vi "generate_DAC_voltages_original.vi"(7 "focus mode?":bool, 8 "derived values":T1, 9 "scan specification":T4={"x amplitude"=0, "x resolution (pixels)"=0, "x offset fly-forward (iterations)"=0, "x offset fly-back (iterations)"=0, "y resolution (nr. of lines)"=0, "y step size"=0, "iterations per pixel"=0, "number of frames"=0, "y offset (pixels)"=0, "number of y-brake lines  (before y-fly-back)"=0, "number y-brake lines (after y-fly-back)"=0, "number of y-fly-back steps"=8, "lines per z step"=0, "number of z/intensity tuples"=0, "number of repetitions (volumes or planes)"=0, "z step size derived"=0, "choose the beginning of z scan"=FALSE, "number of frames (settings)"=0, "FPGA trajectory?"=FALSE}, 10 "counter cluster in":T2, 11 "resonant trigger":bool) -> (0 "acquire?":bool, 1 "fly-back acquisition phase?":bool, 2 "counter cluster out":T2, 3 "DAC voltages":T3 {"ch6" max=4095 step=1; "ch5" max=4095 step=1; "ch4" max=4095 step=1; "ch3" max=4095 step=1; "ch2" max=4095 step=1; "ch1" max=4095 step=1; "ch0" max=4095 step=1})   [LabVIEW 2010]
uses:
  scan_specification_cluster.ctl
  common_typedefs/DAC_voltage_cluster.ctl
  counter_cluster.ctl
  derived_values_cluster.ctl
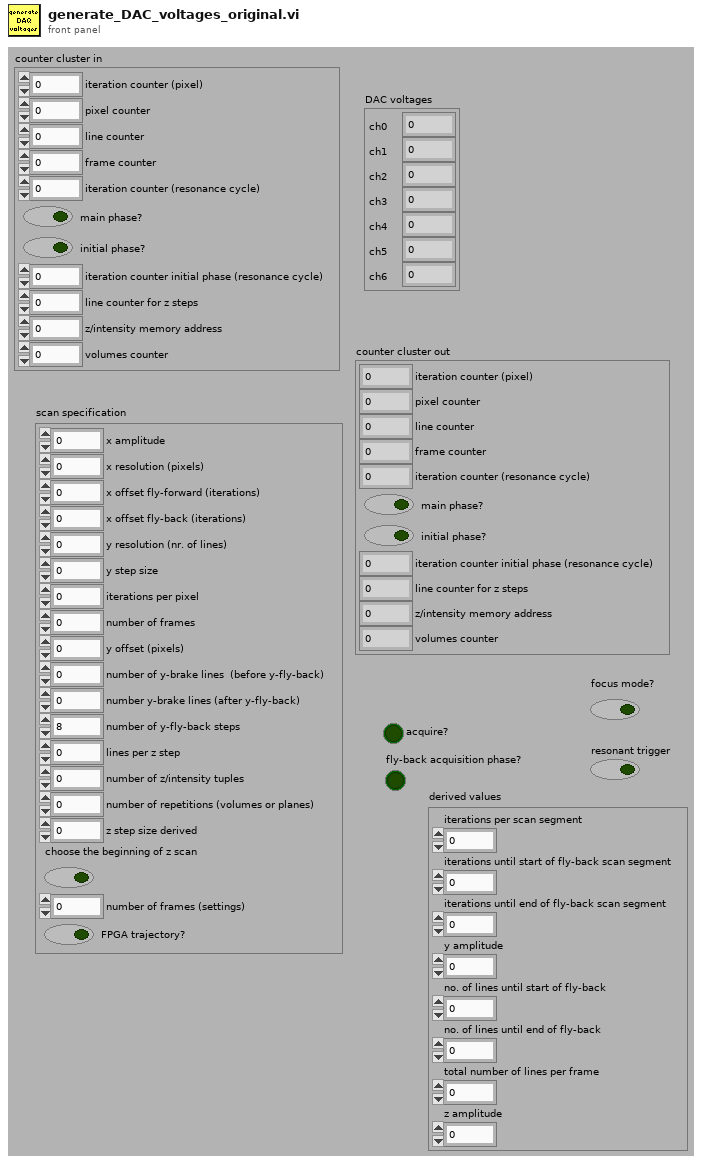
[diagram p1: front panel]
types:
  T1 = typedef "derived_values_cluster.ctl" = cluster{"iterations per scan segment":u16, "iterations until start of fly-back scan segment":u16, "iterations until end of fly-back scan segment":u16, "y amplitude":u16, "no. of lines until start of fly-back":u16, "no. of lines until end of fly-back":u16, "total number of lines per frame ":u16, "z amplitude":u16}
  T2 = typedef "counter_cluster.ctl" = cluster{"iteration counter (pixel)":u16, "pixel counter":u16, "line counter":u16, "frame counter":u16, "iteration counter (resonance cycle)":u16, "main phase?":bool, "initial phase?":bool, "iteration counter initial phase (resonance cycle)":u16, "line counter for z steps":u16, "z/intensity memory address":u32, "volumes counter":u16}
  T3 = typedef "DAC_voltage_cluster.ctl" = cluster{"ch0":u16, "ch1":i16, "ch2":i16, "ch3":u16, "ch4":u16, "ch5":u16, "ch6":u16}
  T4 = typedef "scan_specification_cluster.ctl" = cluster{"x amplitude":u16, "x resolution (pixels)":u16, "x offset fly-forward (iterations)":u16, "x offset fly-back (iterations)":u16, "y resolution (nr. of lines)":u16, "y step size":u16, "iterations per pixel":u16, "number of frames":i32, "y offset (pixels)":u16, "number of y-brake lines  (before y-fly-back)":u16, "number y-brake lines (after y-fly-back)":u16, "number of y-fly-back steps":u16, "lines per z step":u16, "number of z/intensity tuples":u16, "number of repetitions (volumes or planes)":i32, "z step size derived":u16, "choose the beginning of z scan":bool, "number of frames (settings)":i32, "FPGA trajectory?":bool}
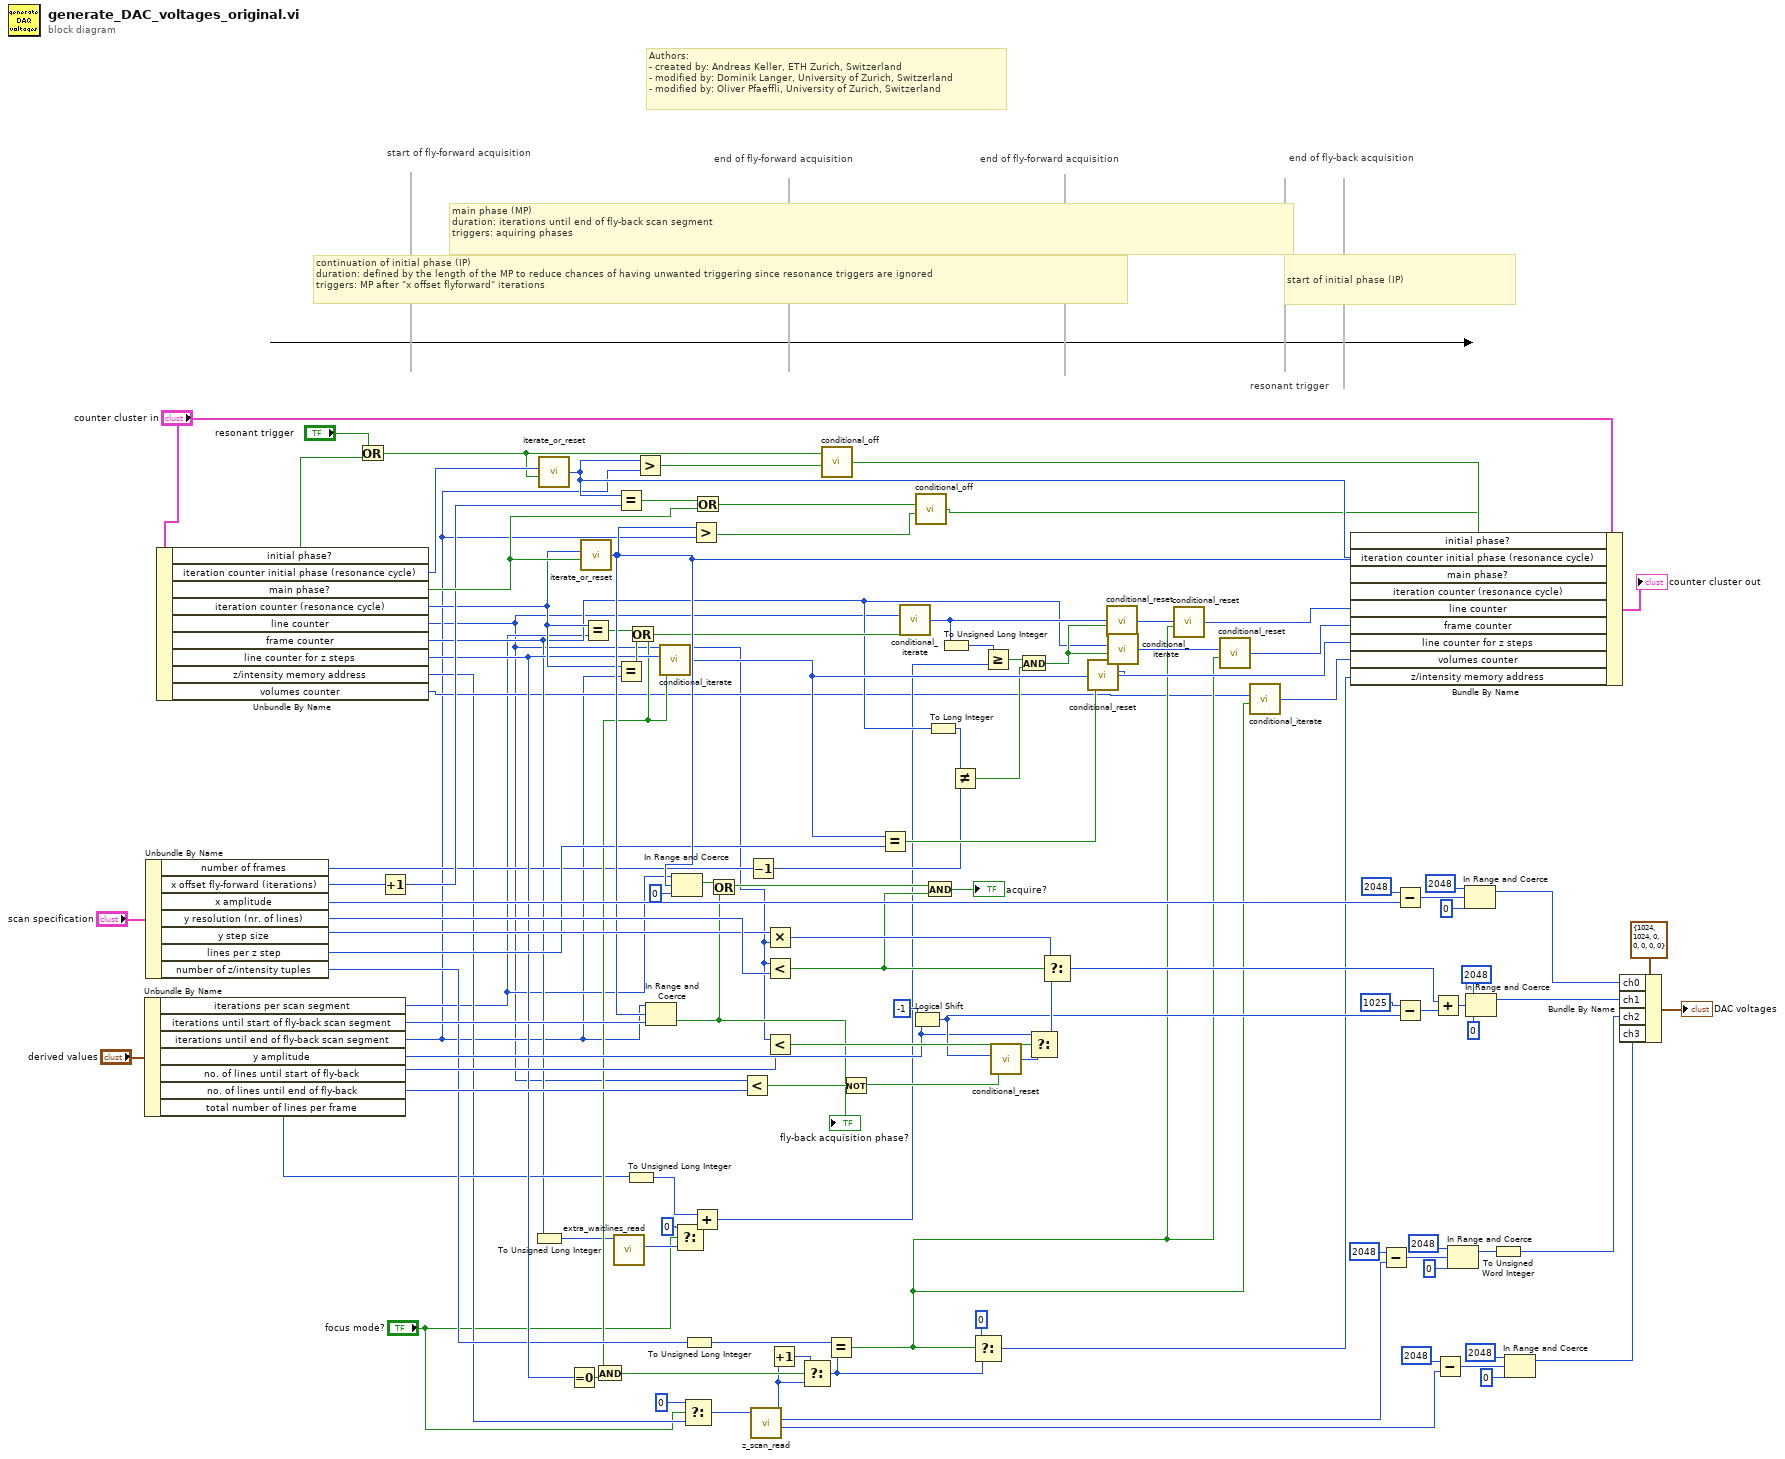
[diagram p0: block diagram]
diagram:
  # "start of initial phase (IP)"
  # "continuation of initial phase (IP)\nduration: defined by the length of the MP to reduce chances of having unwanted triggering since resonance triggers are ignored\ntriggers: MP after \"x offset flyforward\" iterations"
  # "end of fly-back acquisition"
  # "end of fly-forward acquisition"
  # "end of fly-forward acquisition"
  # "start of fly-forward acquisition"
  # "main phase (MP)\nduration: iterations until end of fly-back scan segment\ntriggers: aquiring phases"
  # "resonant trigger"
  # "Authors: \n- created by: Andreas Keller, ETH Zurich, Switzerland\n- modified by: Dominik Langer, University of Zurich, Switzerland\n- modified by: Oliver Pfaeffli, University of Zurich, Switzerland"
  n1 = Unbundle By Name("derived values") -> ("iterations per scan segment"=w5:u16, "iterations until start of fly-back scan segment"=w85:u16, "iterations until end of fly-back scan segment"=w4:u16, "y amplitude"=w69:u16, "no. of lines until start of fly-back"=w68:u16, "no. of lines until end of fly-back"=w84:u16, "total number of lines per frame"=w31:u16)
  n2 = Unbundle By Name("scan specification") -> ("number of frames"=w20:i32, "x offset fly-forward (iterations)"=w67:u16, "x amplitude"=w94:u16, "y resolution (nr. of lines)"=w91:u16, "y step size"=w90:u16, "lines per z step"=w59:u16, "number of z/intensity tuples"=w53:u16)
  n3 = Unbundle By Name("counter cluster in") -> ("initial phase?"=w83:bool, "iteration counter initial phase (resonance cycle)"=w80:u16, "main phase?"=w79:bool, "iteration counter (resonance cycle)"=w63:u16, "line counter"=w2:u16, "frame counter"=w17:u16, "line counter for z steps"=w55:u16, "z/intensity memory address"=w8:u32, "volumes counter"=w10:u16)
  n4 = Or(x="resonant trigger", y=w83) -> (x .or. y?=w76:bool)
  n5 = Increment(x=w67) -> (x+1=w66:u16)
  n6 = To Unsigned Long Integer(number=w17) -> (unsigned 32bit integer=w32:u32)
  n7 = call "iterate_or_reset.vi"("iterate?"=w76, "number in"=w80) -> ("number out"=w64:u16)  [unwired: 4 in]
  n8 = Equal To 0?(x=w55) -> (x = 0?=w38:bool)
  n9 = call "iterate_or_reset.vi"("iterate?"=w79, "number in"=w63) -> ("number out"=w78:u16)  [unwired: 4 in]
  n10 = Equal?(x=w63, y=w5) -> (x = y?=w60:bool)
  n11 = call "extra_waitlines_read.vi"("address extra waitlines IN"=w32) -> ("extra waitline data"=w13:u32)  [unwired: 9 in, 1 out]
  n12 = Equal?(x=w64, y=w66) -> (x = y?=w77:bool)
  n13 = Equal?(x=w63, y=w4) -> (x = y?=w62:bool)
  n14 = To Unsigned Long Integer(number=w31) -> (unsigned 32bit integer=w30:u32)
  n15 = Or(x=w60, y=w62) -> (x .or. y?=w37:bool)
  n16 = And(x=w37, y=w38) -> (x .and. y?=w36:bool)
  n17 = Greater?(x=w64, y=w4) -> (0:w65:bool)
  n18 = In Range and Coerce(upper limit=w4, x=w78, lower limit=w85) -> (In Range?=w61:bool)  [unwired: 1 out]
  "fly-back acquisition phase?" <- w61
  n19 = call "conditional_iterate.vi"("iterate?"=w37, "number in"=w55) -> ("number out"=w56:u16)  [unwired: 4 in]
  n20 = In Range and Coerce(upper limit=w5, x=w78, lower limit=u16 0) -> (In Range?=w106:bool)  [unwired: 1 out]
  n21 = Select(t=u32 0, s="focus mode?", f=w13) -> (s? t:f=w12:u32)
  n22 = Select(t=u32 0, s="focus mode?", f=w8) -> (s? t:f=w7:u32)
  n23 = To Unsigned Long Integer(number=w53) -> (unsigned 32bit integer=w52:u32)
  n24 = Greater?(x=w78, y=w4) -> (0:w74:bool)
  n25 = Add(x=w30, y=w12) -> (x+y=w14:u32)
  n26 = Or(x=w77, y=w79) -> (x .or. y?=w73:bool)
  n27 = Or(x=w106, y=w61) -> (x .or. y?=w89:bool)
  n28 = Less?(x=w2, y=w84) -> (x < y?=w87:bool)
  n29 = Decrement(x=w20) -> (x-1=w19:i32)
  n30 = call "z_scan_read.vi"("address in"=w7) -> ("intensity"=w35:u16, "z-value"=w33:i16, "address out"=w34:u32)  [unwired: 8 in]
  n31 = Multiply(x=w90, y=w2) -> (x*y=w112:u16)
  n32 = Less?(x=w2, y=w91) -> (x < y?=w88:bool)
  n33 = Less?(x=w2, y=w68) -> (x < y?=w114:bool)
  n34 = Increment(x=w34) -> (x+1=w54:u32)
  n35 = Select(t=w54, s=w36, f=w34) -> (s? t:f=w51:u32)
  n36 = call "conditional_off.vi"("switch off?"=w65, "boolean in"=w76) -> ("boolean out"=w75:bool)  [unwired: 4 in]
  n37 = Equal?(x=w52, y=w51) -> (x = y?=w15:bool)
  n38 = Not(x=w87) -> (.not. x?=w71:bool)
  n39 = Equal?(x=w56, y=w59) -> (x = y?=w57:bool)
  n40 = call "conditional_iterate.vi"("iterate?"=w37, "number in"=w2) -> ("number out"=w29:u16)  [unwired: 4 in]
  n41 = Logical Shift(y=i16 -1 ("n"), x=w69) -> (x << y=w72:u16)
  n42 = call "conditional_off.vi"("switch off?"=w74, "boolean in"=w73) -> ("boolean out"=w1:bool)  [unwired: 4 in]
  n43 = And(x=w89, y=w88) -> (x .and. y?=→"acquire?":bool)
  n44 = To Long Integer(number=w17) -> (32bit integer=w16:i32)
  n45 = To Unsigned Long Integer(number=w29) -> (unsigned 32bit integer=w28:u32)
  n46 = Not Equal?(x=w16, y=w19) -> (x != y?=w18:bool)
  n47 = Select(t=u32 0, s=w15, f=w51) -> (s? t:f=w27:u32)
  n48 = Greater Or Equal?(x=w28, y=w14) -> (x >= y?=w22:bool)
  n49 = call "conditional_reset.vi"("reset?"=w71, "number in"=w72) -> ("number out"=w70:u16)  [unwired: 4 in]
  n50 = And(x=w22, y=w18) -> (x .and. y?=w21:bool)
  n51 = Select(t=w69, s=w114, f=w70) -> (s? t:f=w113:u16)
  n52 = Select(t=w112, s=w88, f=w113) -> (s? t:f=w92:u16)
  n53 = call "conditional_reset.vi"("reset?"=w57, "number in"=w56) -> ("number out"=w58:u16)  [unwired: 4 in]
  n54 = call "conditional_reset.vi"("reset?"=w21, "number in"=w29) -> ("number out"=w23:u16)  [unwired: 4 in]
  n55 = call "conditional_iterate.vi"("iterate?"=w21, "number in"=w17) -> ("number out"=w25:u16)  [unwired: 4 in]
  n56 = call "conditional_reset.vi"("reset?"=w15, "number in"=w23) -> ("number out"=w3:u16)  [unwired: 4 in]
  n57 = call "conditional_reset.vi"("reset?"=w15, "number in"=w25) -> ("number out"=w26:u16)  [unwired: 4 in]
  n58 = call "conditional_iterate.vi"("iterate?"=w15, "number in"=w10) -> ("number out"=w24:u16)  [unwired: 4 in]
  n59 = Bundle By Name(cluster="counter cluster in", "initial phase?"=w75, "iteration counter initial phase (resonance cycle)"=w64, "main phase?"=w1, "iteration counter (resonance cycle)"=w78, "line counter"=w3, "frame counter"=w26, "line counter for z steps"=w58, "volumes counter"=w24, "z/intensity memory address"=w27) -> (→"counter cluster out":T2)
  n60 = Subtract(x=i16 2048, y=w33) -> (x-y=w43:i16)
  n61 = Subtract(x=u16 2048, y=w94) -> (x-y=w98:u16)
  n62 = Subtract(x=u16 1025, y=w72) -> (x-y=w105:u16)
  n63 = Add(x=w92, y=w105) -> (x+y=w101:u16)
  n64 = Subtract(x=u16 2048, y=w35) -> (x-y=w47:u16)
  n65 = In Range and Coerce(upper limit=i16 2048, x=w43, lower limit=i16 0) -> (coerced(x)=w40:i16)  [unwired: 1 out]
  n66 = In Range and Coerce(upper limit=u16 2048, x=w98, lower limit=u16 0) -> (coerced(x)=w97:u16)  [unwired: 1 out]
  n67 = In Range and Coerce(upper limit=u16 2048, x=w101, lower limit=u16 0) -> (coerced(x)=w100:u16)  [unwired: 1 out]
  n68 = To Unsigned Word Integer(number=w40) -> (unsigned 16bit integer=w39:u16)
  n69 = In Range and Coerce(upper limit=u16 2048, x=w47, lower limit=u16 0) -> (coerced(x)=w45:u16)  [unwired: 1 out]
  n70 = Bundle By Name(cluster=T3 {"ch0"=1024, "ch1"=1024, "ch2"=0, "ch3"=0, "ch4"=0, "ch5"=0, "ch6"=0} ("DAC voltage"), "ch0"=w97, "ch1"=w100, "ch2"=w39, "ch3"=w45) -> (→"DAC voltages":T3)
